vi "Update Status.vi"(7 "Status Listbox":refnum<vi>, 8 "error in (no error)":errorcluster, 9 "Component":string, 10 "Time":timestamp, 11 "Status":string) -> (0 "error out":errorcluster, 3 "dup Status":string)   [LabVIEW 2024]
doc: "Updates the running status in the log list."
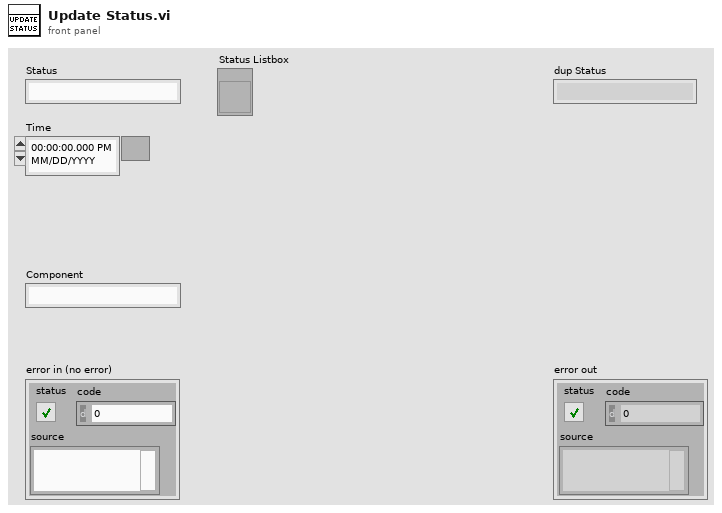
[diagram p1: front panel]
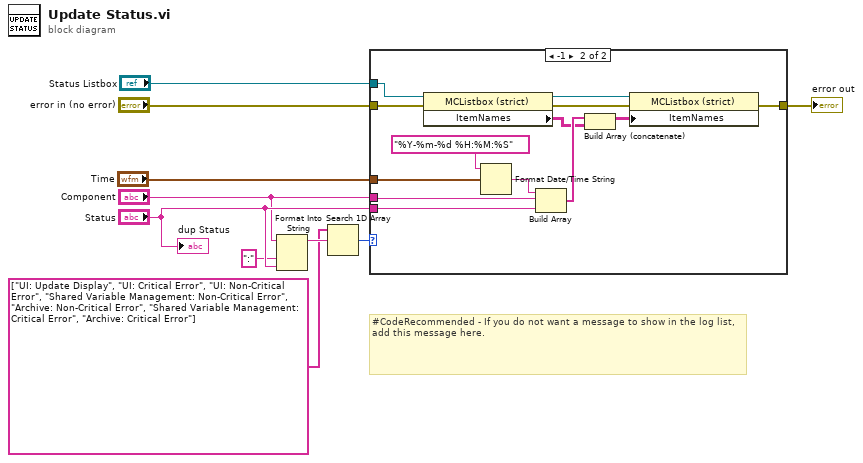
[diagram p0: block diagram]
diagram:
  # "#CodeRecommended - If you do not want a message to show in the log list, add this message here."
  n1 = Format Into String(initial string="Component", ":" ("input 1"), "Status") -> (resulting string=w4:string)  [unwired: 2 in, 1 out]
  n2 = Search 1D Array(1D array=string[] ["UI: Update Display", "UI: Critical Error", "UI: Non-Critical Error", "Shared Variable Management: Non-Critical Error", "Archive: Non-Critical Error", "Shared Variable Management: Critical Error", "Archive: Critical Error"], element=w4) -> (index of element=w1:i32)  [unwired: 1 in]
  n3 = case shown="-1" w1 {
    tunnel: [w11 w15] -> w9
    tunnel: "error in (no error)" -> [w11 w21]
    tunnel: "Status" -> [_ w20]
    tunnel: "Component" -> [_ w18]
    tunnel: "Time" -> [_ w17]
    tunnel: "Status Listbox" -> [_ w16]
    frame Default {
    }
    frame -1 {
      n4 = property class="MCListbox (strict)"(reference=w16, error in=w21) -> (reference out=w24:refnum<vi>, error out=w23:errorcluster, "ItemNames"=w13:string[][])
      n5 = Format Date/Time String(time format string (%c)="%Y-%m-%d %H:%M:%S", seconds (now)=w17) -> (date/time string=w19:string)  [unwired: 1 out]
      n6 = Build Array(w19, w18, w20) -> (w14:string[])
      n7 = Build Array (concatenate)(w14, w13) -> (w12:string[][])
      n8 = property class="MCListbox (strict)"(reference=w24, error in=w23, "ItemNames"=w12) -> (error out=w15:errorcluster)  [unwired: 1 out]
    }
  }
  "error out" <- w9
  "dup Status" <- "Status"
